vi "Visa Read data.vi"(8 "错误输入（无错误）":errorcluster, 11 "VISA Name":T1={"VISA"="", "baud rate"=9600, "data bits"=8, "parity"=enum."None", "stop bits"=10, "flow control"=0} {"flow control" items=["None", "XON/XOFF", "RTS/CTS", "XON/XOFF & RTS/CTS", "DTR/DSR", "XON/XOFF & DTR/DSR"]; "stop bits" items=["1.0"=10, "1.5"=15, "2.0"=20]}) -> (0 "error out":errorcluster, 1 "State":bool, 2 "trimmed string":string caption="Code", 3 "VISA Name out":T1={"VISA"="", "baud rate"=9600, "data bits"=8, "parity"=enum."None", "stop bits"=10, "flow control"=0} {"flow control" items=["None", "XON/XOFF", "RTS/CTS", "XON/XOFF & RTS/CTS", "DTR/DSR", "XON/XOFF & DTR/DSR"]; "stop bits" items=["1.0"=10, "1.5"=15, "2.0"=20]})   [LabVIEW 2014]
uses:
  <vilib>/Utility/error.llb/whitespace.ctl
  Ctr/VISA Ctr.ctl
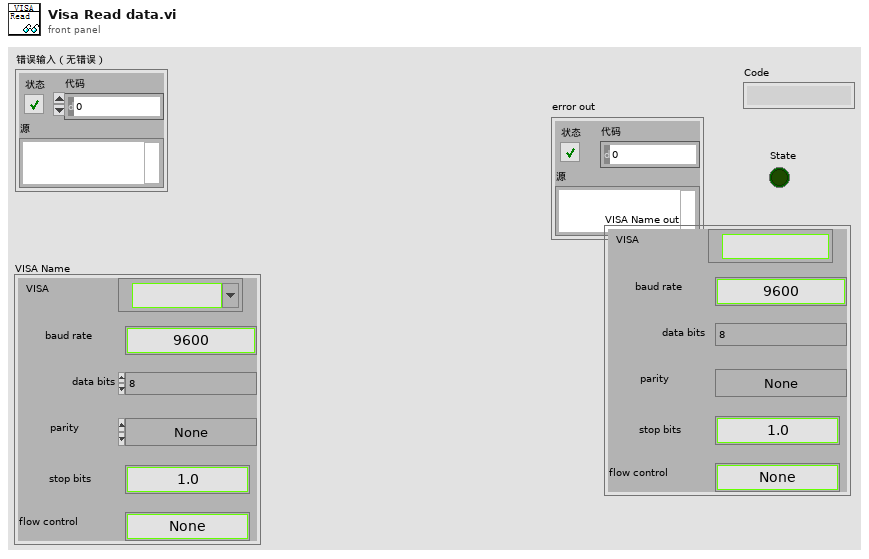
[diagram p1: front panel]
types:
  T1 = typedef "VISA Ctr.ctl" = cluster{"VISA":refnum<visa-resource-name>, "baud rate":u32, "data bits":u16, "parity":enum16{"None", "Odd", "Even", "Mark", "Space"}, "stop bits":u16, "flow control":u16}
  T2 = typedef "whitespace.ctl" = u16
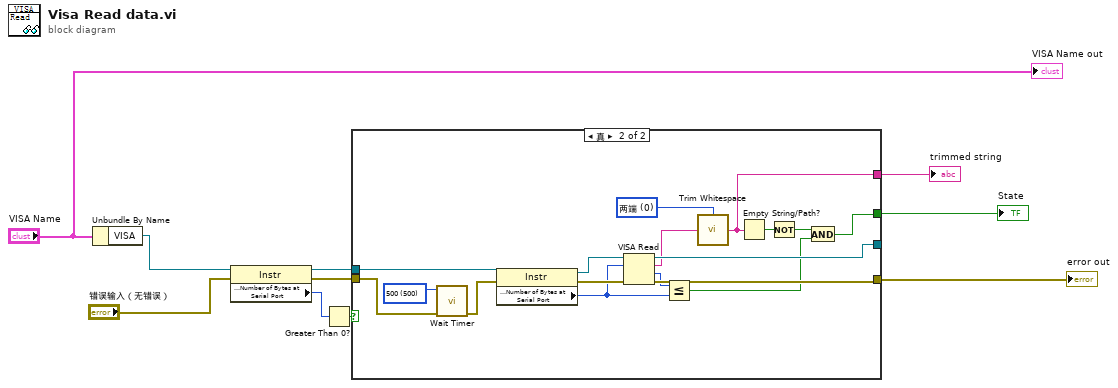
[diagram p0: block diagram]
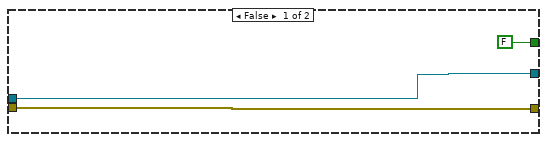
[diagram p2: hidden frame]
diagram:
  n1 = Unbundle By Name("VISA Name") -> ("VISA"=w2:refnum<visa-resource-name>)
  n2 = property class="Instr"(reference=w2, error in="错误输入（无错误）") -> (reference out=w6:refnum<visa-resource-name>, error out=w7:errorcluster, "Serial Settings:Number of Bytes at Serial Port"=w9:u32)
  n3 = Greater Than 0?(x=w9) -> (x > 0?=w8:bool)
  n4 = case shown="真" w8 {
    tunnel: w7 -> [w13 w30]
    tunnel: w6 -> [w12 w28]
    tunnel: [w13 w24] -> w4
    tunnel: [w12 w23] -> _
    tunnel: [FALSE w15] -> w5
    tunnel: [_ w14] -> w1
    frame False {
    }
    frame True {
      w19 = T2 0 items=["两端", "字符串首端", "字符串末端"] ("location (both)")
      w29 = u16 500 items=["10"=10, "20"=20, "50"=50, "80"=80, "100"=100, "200"=200, "300"=300, "400"=400, "500"=500, "600"=600, "700"=700, "800"=800, "900"=900, "1000"=1000] ("Dely")
      n5 = call "Wait Timer.vi"("error in (no error)"=w30, "Dely"=w29) -> ("error out"=w27:errorcluster)  [unwired: 8 in, 1 out]
      n6 = property class="Instr"(reference=w28, error in=w27) -> (reference out=w25:refnum<visa-resource-name>, error out=w26:errorcluster, "Serial Settings:Number of Bytes at Serial Port"=w21:u32)
      n7 = VISA Read(VISA resource name=w25, byte count=w21, error in (no error)=w26) -> (VISA resource name out=w23:refnum<visa-resource-name>, read buffer=w20:string, return count=w22:u32, error out=w24:errorcluster)
      n8 = Less Or Equal?(x=w22, y=w21) -> (x <= y?=w16:bool)
      n9 = call <vilib>:"Trim Whitespace.vi"("string"=w20, "location (both)"=w19) -> ("trimmed string"=w14:string)
      n10 = Empty String/Path?(string/path=w14) -> (empty?=w18:bool)
      n11 = Not(x=w18) -> (.not. x?=w17:bool)
      n12 = And(x=w17, y=w16) -> (x .and. y?=w15:bool)
    }
  }
  "State" <- w5
  "error out" <- w4
  "trimmed string" <- w1
  "VISA Name out" <- "VISA Name"
